vi "Host Read Characters From File.vi"(0 "file path":path, 1 "prompt":string, 5 "start path (Not A Path)":path, 7 "default name":string, 9 "[pattern]":string, 11 "number of characters (all:-1)":i32=-1, 12 "convert eol? (no:F)":bool, 13 "start of read offset (chars.: 0)":i32, 14 "RT Reference":refnum<vi>) -> (4 "new file path (NotAPath if cancelled)":path, 6 "character string":string, 8 "mark after read (chars.)":i32, 10 "EOF?":bool, 15 "error out 2":errorcluster)   [LabVIEW 2023]
doc: "Reads a specified number of characters from a byte stream file beginning at a specified character offset."
panel:
  out "error out":errorcluster
  in  "error":errorcluster
  in  "type specifier VI Refnum (for type only)":refnum<vi>
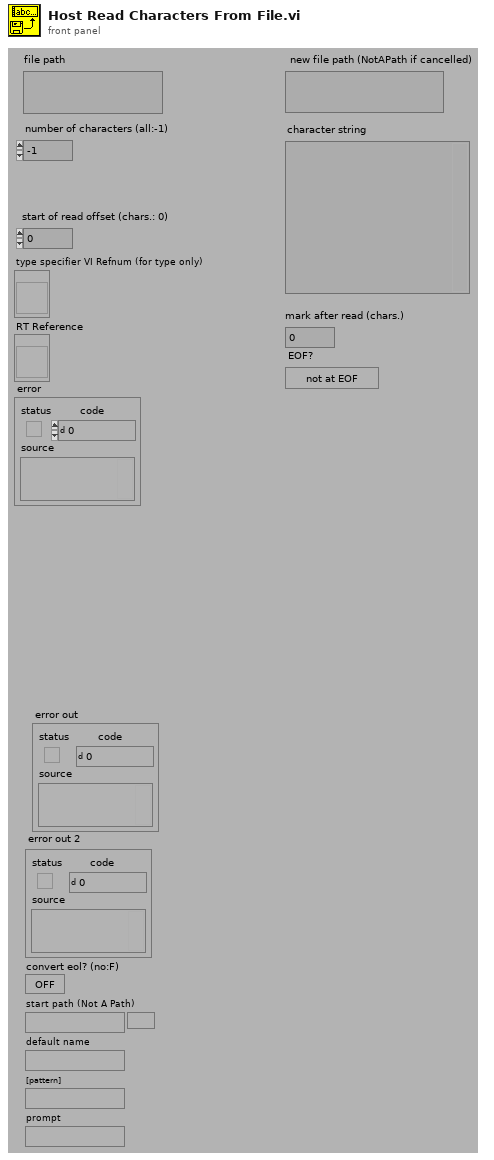
[diagram p1: front panel]
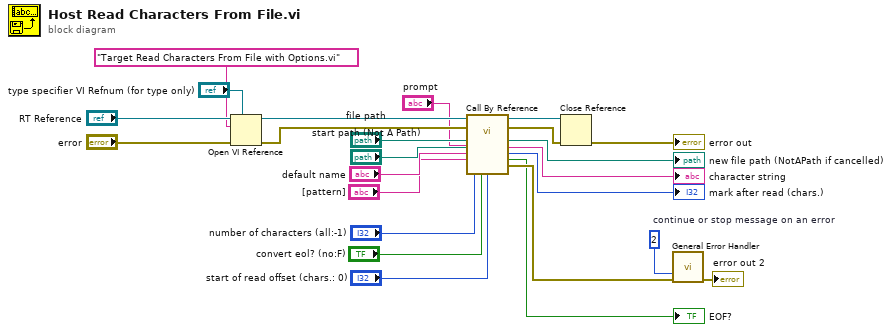
[diagram p0: block diagram]
diagram:
  w24 = u16 2  # continue or stop message on an error
  n1 = Open VI Reference(type specifier VI Refnum (for type only)="type specifier VI Refnum (for type only)", application reference (local)="RT Reference", vi path="Target Read Characters From File with Options.vi", error in (no error)="error") -> (vi reference=w23:refnum<vi>, error out=w22:errorcluster)  [unwired: 2 in]
  n2 = call-by-ref "?"(reference=w23, error in=w22, "file path (dialog if empty)"="file path", "prompt"="prompt", "start path (Not A Path)"="start path (Not A Path)", "default name"="default name", "[pattern]"="[pattern]", "number of characters (all:-1)"="number of characters (all:-1)", "convert eol? (no:F)"="convert eol? (no:F)", "start of read offset (chars.: 0)"="start of read offset (chars.: 0)") -> (reference out=w15:refnum<vi>, error out=w14:errorcluster, "new file path (NotAPath if cancelled)"=→"new file path (NotAPath if cancelled)":path, "character string"=→"character string":string, "mark after read (chars.)"=→"mark after read (chars.)":i32, "EOF?"=→"EOF?":bool, 15:"error out"=w10:errorcluster)  [unwired: 3 in]
  n3 = Close Reference(reference=w15, error in (no error)=w14) -> (error out=→"error out":errorcluster)
  n4 = call <vilib>:"General Error Handler.vi"("type of dialog (OK msg:1)"=w24, "error in (no error)"=w10) -> ("error out"=→"error out 2":errorcluster)  [unwired: 9 in, 4 out]
